vi "Execute Free Label To VI Description.vi"(6 "Mouse Position":T1, 8 "User VI Ref":refnum<vi>, 9 "Menu Item Tag Suffix":string, 10 "Remaining Items":refnum<vi>[](array[refnum]), 11 "Affected Items":cluster{"Free Labels (Comments)":refnum<vi>[]}) -> (0 "Fail transaction?":bool)   [LabVIEW 2022 SP3]
doc: "This VI is part of a plug-in for modifying the LabVIEW shortcut menus. This is the execute VI which is called when the shortcut menu is chosen by the user. It performs the action of the selected menu item."
uses:
  <vilib>/Utility/miscctls.llb/LVPositionTypeDef.ctl
panel:
  # "All controls on this panel except \"Affected Items\" have been locked to prevent accidental edits. Changing the control names or types, other than the elements of the \"Affected Items\" cluster will make the VI unusable as a menu plugin.\n\nSee Context Help for each control for details about its use."
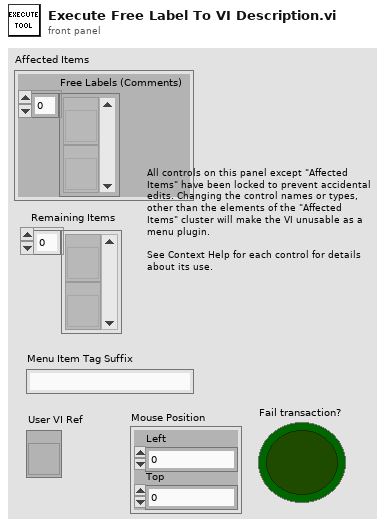
[diagram p1: front panel]
types:
  T1 = typedef "LVPositionTypeDef.ctl" = cluster{"Left":i32, "Top":i32}
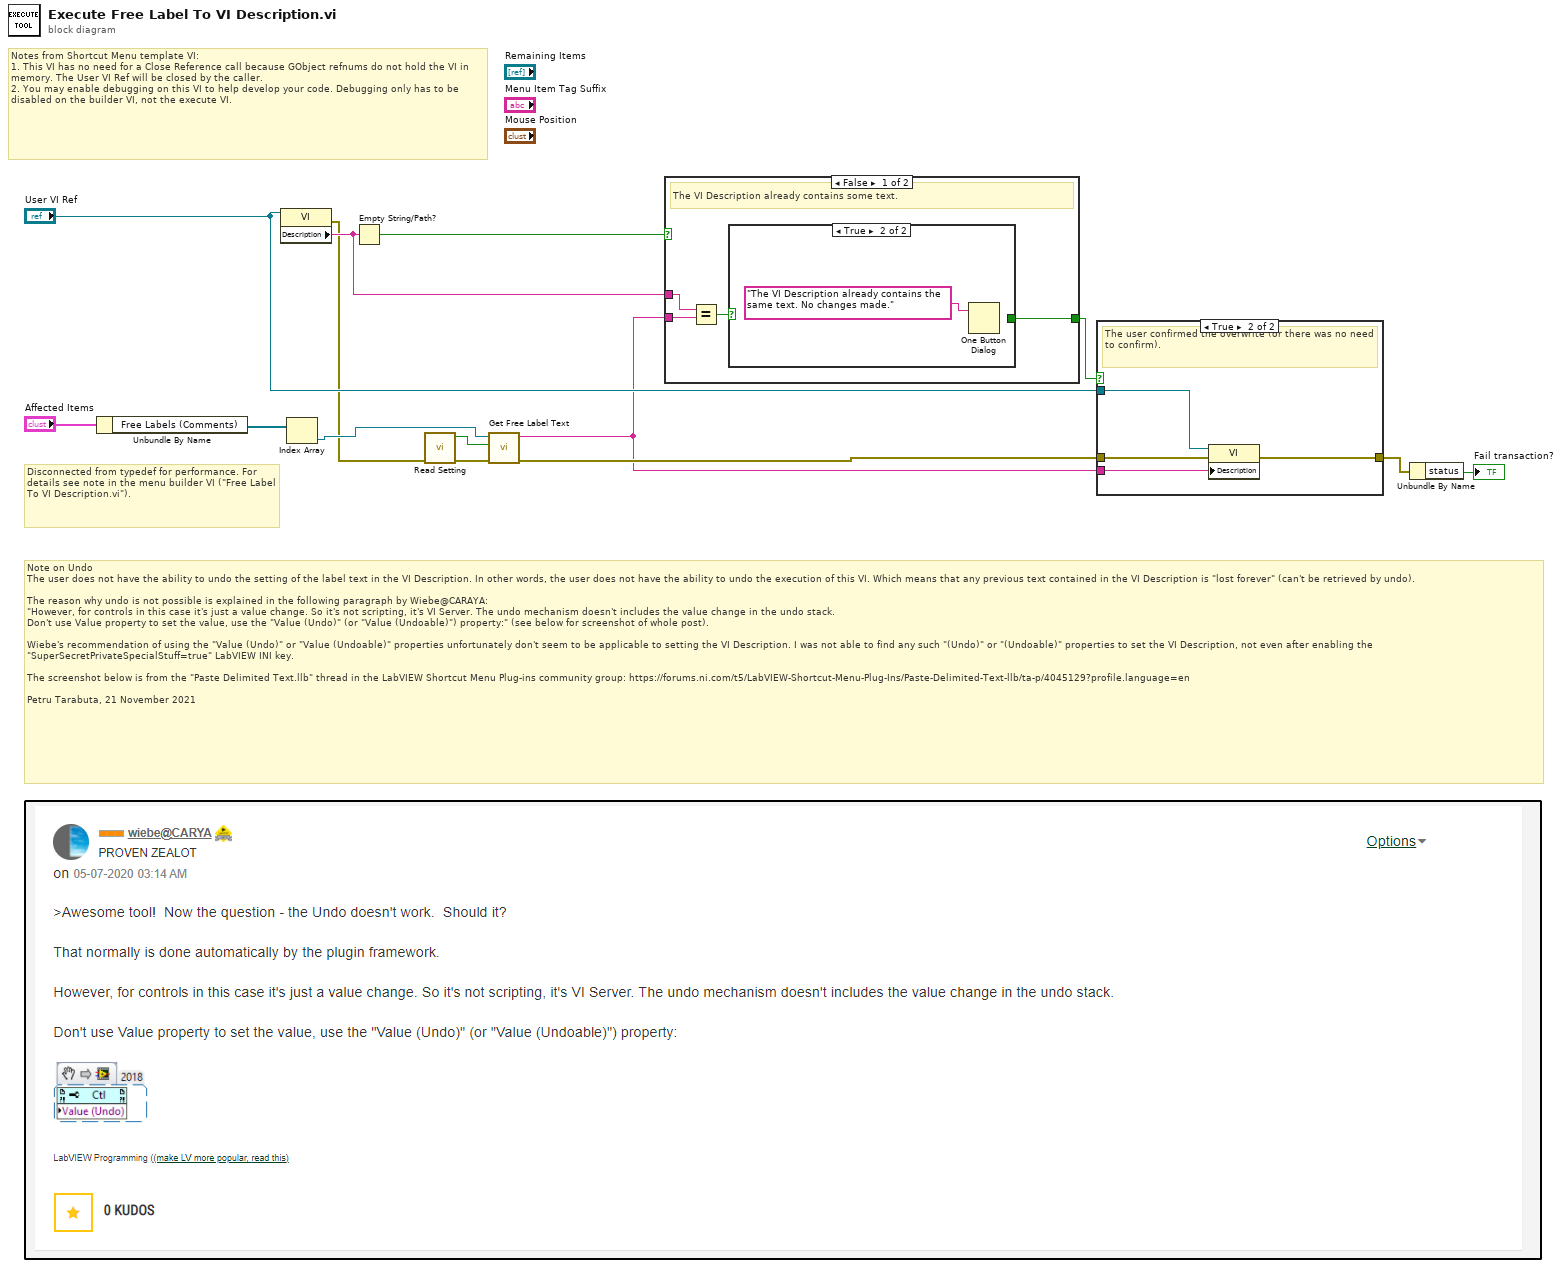
[diagram p0: block diagram]
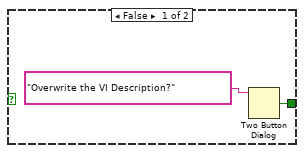
[diagram p2: hidden frame]
diagram:
  # "Disconnected from typedef for performance. For details see note in the menu builder VI (\"Free Label To VI Description.vi\")."
  # "Note on Undo\nThe user does not have the ability to undo the setting of the label text in the VI Description. In other words, the user does not have the ability to undo the execution of this VI. Which means that any previous text contained in the VI Description is \"lost forever\" (can't be retrieved by undo).\n\nThe reason why undo is not possible is explained in the following paragraph by Wiebe@CARAYA: \n\"However, for controls in this case it's just a value change. So it's not scripting, it's VI Server. The undo mechanism doesn't includes the value change in the undo stack.\nDon't use Value property to set the value, use the \"Value (Undo)\" (or \"Value (Undoable)\") property:\" (see below for screenshot of whole post).\n\nWiebe's recommendation of using the \"Value (Undo)\" or \"Value (Undoable)\" properties unfortunately don't seem to be applicable to setting the VI Description. I was not able to find any such \"(Undo)\" or \"(Undoable)\" properties to set the VI Description, not even after enabling the \"SuperSecretPrivateSpecialStuff=true\" LabVIEW INI key.\n\nThe screenshot below is from the \"Paste Delimited Text.llb\" thread in the LabVIEW Shortcut Menu Plug-ins community group: https://forums.ni.com/t5/LabVIEW-Shortcut-Menu-Plug-Ins/Paste-Delimited-Text-llb/ta-p/4045129?profile.language=en\n\nPetru Tarabuta, 21 November 2021"
  # "Notes from Shortcut Menu template VI:\n1. This VI has no need for a Close Reference call because GObject refnums do not hold the VI in memory. The User VI Ref will be closed by the caller.\n2. You may enable debugging on this VI to help develop your code. Debugging only has to be disabled on the builder VI, not the execute VI."
  n1 = Unbundle By Name("Affected Items") -> ("Free Labels (Comments)"=w13:refnum<vi>[])
  n2 = property class="VI"(reference="User VI Ref") -> (error out=w5:errorcluster, "Description"=w6:string)  [unwired: 1 in, 1 out]
  n3 = Index Array(array=w13) -> (element=w14:refnum<vi>)  [unwired: 1 in]
  n4 = Empty String/Path?(string/path=w6) -> (empty?=w11:bool)
  n5 = call "Read Setting.vi"("Error In"=w5) -> ("Error Out"=w2:errorcluster, "Process Bold Characters?"=w1:bool)  [unwired: 9 in]
  n6 = call "Get Free Label Text.vi"("Error In"=w2, "Process Bold Characters?"=w1, "Free Label Ref"=w14) -> ("Error Out"=w4:errorcluster, "VI Description Text"=w3:string)  [unwired: 6 in, 1 out]
  n7 = case shown="False" w11 {
    selector: w11 -> [_ w22]
    tunnel: [w18 w22] -> w10
    tunnel: w3 -> [w17 _]
    tunnel: w6 -> [w16 _]
    frame False {
      # "The VI Description already contains some text."
      n8 = Equal?(x=w16, y=w17) -> (x = y?=w15:bool)
      n9 = case shown="True" w15 {
        tunnel: [w19 _] -> w18
        frame False {
          n10 = Two Button Dialog(message="Overwrite the VI Description?") -> (T button?=w19:bool)  [unwired: 2 in]
        }
        frame True {
          n11 = One Button Dialog(message="The VI Description already contains the same text. No changes made.") -> ()  [unwired: 1 in, 1 out]
        }
      }
    }
    frame True {
      # "The VI Description was empty before the user pressed \"Set as VI Description\""
    }
  }
  n12 = case shown="True" w10 {
    tunnel: w4 -> [w23 w24]
    tunnel: "User VI Ref" -> [_ w26]
    tunnel: [w23 w27] -> w7
    tunnel: w3 -> [_ w25]
    frame False {
      # "Do nothing."
      # "The user did not confirm. Might have changed their mind or might have pressed the menu item accidentally."
    }
    frame True {
      # "The user confirmed the overwrite (or there was no need to confirm)."
      n13 = property class="VI"(reference=w26, error in=w24, "Description"=w25) -> (error out=w27:errorcluster)  [unwired: 1 out]
    }
  }
  n14 = Unbundle By Name(w7) -> ("status"=→"Fail transaction?":bool)
